vi "LV2OO Style Global_Static.vi"(4 "error in (no error)":errorcluster, 7 "Action in":refnum<class "Action.lvclass">) -> (0 "error out":errorcluster, 3 "Action out":refnum<class "Action.lvclass">)   [LabVIEW 2014]
uses:
  Core Components/Action/Action.lvclass
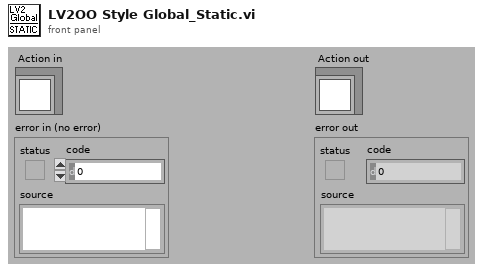
[diagram p1: front panel]
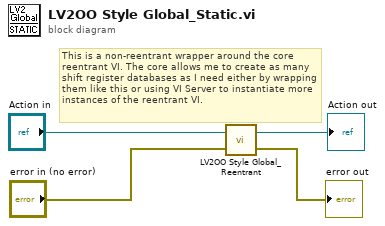
[diagram p0: block diagram]
diagram:
  # "This is a non-reentrant wrapper around the core reentrant VI. The core allows me to create as many shift register databases as I need either by wrapping them like this or using VI Server to instantiate more instances of the reentrant VI."
  n1 = call "LV2OO Style Global_Reentrant.vi"("error in (no error)"="error in (no error)", "Action in"="Action in") -> ("error out"=→"error out":errorcluster, "Action out"=→"Action out":refnum<class "Action.lvclass">)
